vi "Charge and Discharge.vi"(8 "TDMS File Path In":string, 9 "Voltage":dbl=1.5, 10 "Initial Capacity  (mAh)":dbl=2350.0, 11 "Cycle":i32) -> (0 "TDMS File Path":string, 1 "Passed":bool, 2 "Energy (Wh)":dbl, 3 "Capacity (mAh)":dbl)   [LabVIEW 2020]
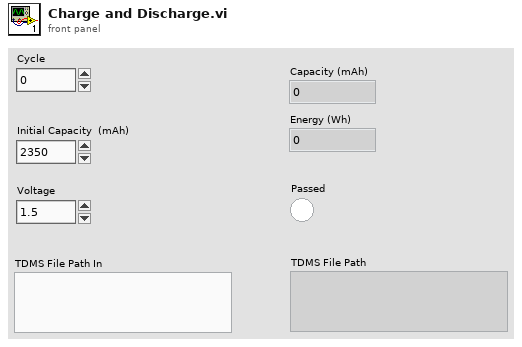
[diagram p1: front panel]
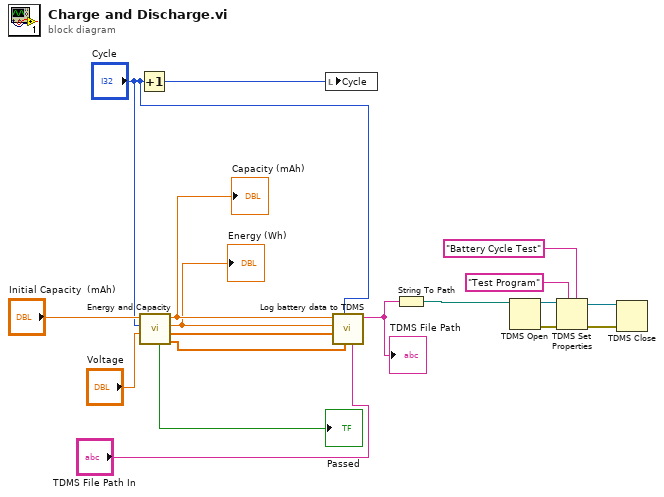
[diagram p0: block diagram]
diagram:
  n1 = Increment(x="Cycle") -> (x+1=w16:i32)
  n2 = call "Energy and Capacity.vi"("Voltage"="Voltage", "Cycle"="Cycle", "Initial Capacity  (mAh) in"="Initial Capacity  (mAh)") -> ("Current (mA)"=w9:dbl[], "Voltage (V)"=w11:dbl[], "Energy (Wh)"=w14:dbl, "Capacity  (mAh)"=w15:dbl, "Pass"=→"Passed":bool)  [unwired: 4 in]
  "Energy (Wh)" <- w14
  "Capacity (mAh)" <- w15
  n3 = local write "Cycle"(w16) -> ()
  n4 = call "Log battery data to TDMS.vi"("TDMS File Path In"="TDMS File Path In", "Current (mA)"=w9, "Cycle"="Cycle", "Voltage (V)"=w11, "Energy (Wh)"=w14, "Capacity  (mAh)"=w15) -> ("TDMS File Path Out"=w7:string)  [unwired: 5 in]
  "TDMS File Path" <- w7
  n5 = String To Path(string=w7) -> (path=w6:path)
  n6 = TDMS Open(11:w6) -> (0:w5:errorcluster, 3:w8:refnum<k34>)  [unwired: 6 in]
  n7 = TDMS Set Properties(5:"Battery Cycle Test", 7:"Test Program", 8:w5, 11:w8) -> (0:w1:errorcluster, 3:w2:refnum<k34>)  [unwired: 2 in, 2 out]
  n8 = TDMS Close(8:w1, 11:w2) -> ()  [unwired: 2 out]
